vi "BRig_RT_comm_webdav_testConnect.vi"(10 "input_password":string, 11 "input_username":string="Paul Jonak") -> (2 "output_Iconnected":bool)   [LabVIEW 2014]
uses:
  <vilib>/WebDAVClient/NI_WebDAV.lvlib
panel:
  out "error out":errorcluster
  out "output_code":u8
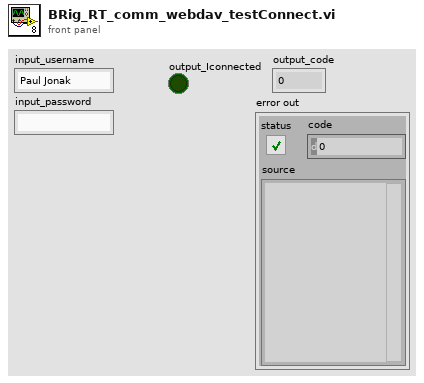
[diagram p1: front panel]
types:
  T1 = typedef "NI_WebDAV.lvlib/SessionHandle.ctl" = refnum<k1>
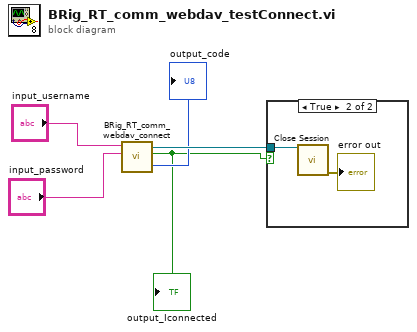
[diagram p0: block diagram]
diagram:
  n1 = call "BRig_RT_comm_webdav_connect.vi"("input_password"="input_password", "input_username"="input_username") -> ("output_Iconnected"=w1:bool, "output_hSession"=w4:T1, "output_code"=→"output_code":u8)  [unwired: 6 in, 1 out]
  "output_Iconnected" <- w1
  n2 = case shown="True" w1 {
    tunnel: w4 -> [_ w7]
    frame False {
    }
    frame True {
      n3 = call <vilib>:"Close Session.vi"("session handle"=w7) -> ("error out"=→"error out":errorcluster)  [unwired: 14 in]
    }
  }
